vi "显示测试结果-左上角-拍照螺杆.vi"(8 "显示坐标":cluster{dbl, "Numeric":dbl}[](array[cluster])=[{100.0, "Numeric"=300.0}, {100.0, "Numeric"=400.0}, {100.0, "Numeric"=500.0}, {100.0, "Numeric"=600.0}, {100.0, "Numeric"=700.0}, {100.0, "Numeric"=800.0}, {100.0, "Numeric"=900.0}, {100.0, "Numeric"=1000.0}, {100.0, "Numeric"=1100.0}], 9 "量测项目名称":string[](array[string]), 10 "显示数据":dbl[](array[numeric]), 11 "Img输入":T1) -> ()   [LabVIEW 2014]
uses:
  <vilib>/vision/Image Controls.llb/IMAQ Image.ctl
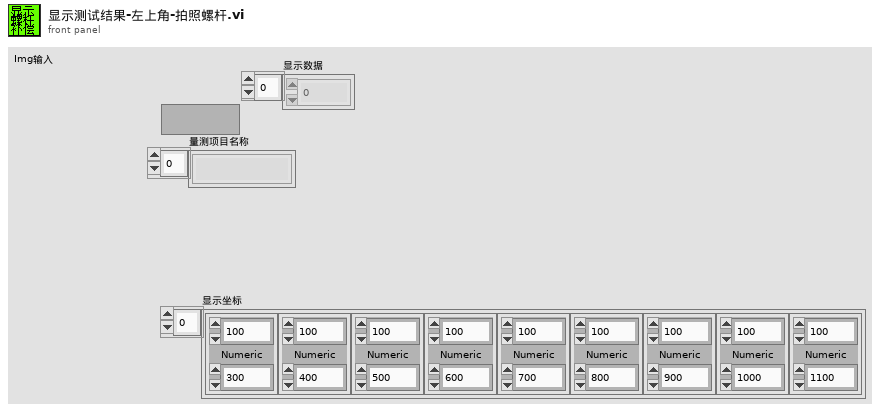
[diagram p1: front panel]
types:
  T1 = typedef "IMAQ Image.ctl" = refnum<image>
  T2 = cluster{"Desired Font (Application)":enum16{"User-specified Font", "Application Font", "System Font", "Dialog Font"}, "[User-specified Font]":cluster{"Font Name":string, "Size":i16, "Strikeout?":bool, "Italic?":bool, "Underline?":bool, "Outline?":bool, "Shadow?":bool, "Bold?":bool, "Rotation Angle":dbl}, "Horizontal Alignment":i16, "Vertical Alignment":i16}
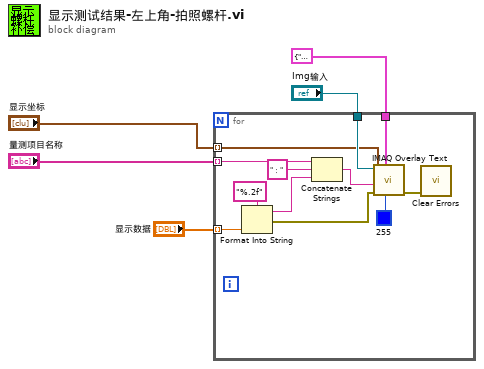
[diagram p0: block diagram]
diagram:
  n1 = for {
    tunnel: "Img输入" -> [w17]
    tunnel: "显示数据" -> [w16] mode=indexing
    tunnel: "显示坐标" -> [w15] mode=indexing
    tunnel: T2 {"Desired Font (Application)"=enum."User-specified Font", "[User-specified Font]"={"Font Name"="", "Size"=80, "Strikeout?"=FALSE, "Italic?"=FALSE, "Underline?"=FALSE, "Outline?"=FALSE, "Shadow?"=FALSE, "Bold?"=FALSE, "Rotation Angle"=0.0}, "Horizontal Alignment"=0, "Vertical Alignment"=0} ("Font, Size & Style") -> [w14]
    tunnel: "量测项目名称" -> [w10] mode=indexing
    n2 = Format Into String(format string="%.2f" ("格式字符串"), w16) -> (resulting string=w8:string, error out=w12:errorcluster)  [unwired: 2 in]
    n3 = Concatenate Strings(w10, "：" ("字符串"), w8) -> (w9:string)
    n4 = call "IMAQ Overlay Text"("Text Color (black)"=u32 255, "Font, Size & Style"=w14, "error in (no error)"=w12, "String"=w9, "Origin"=w15, "Image"=w17) -> ("error out"=w11:errorcluster)  [unwired: 4 in, 1 out]
    n5 = call <vilib>:"Clear Errors.vi"("error in (no error)"=w11) -> ()  [unwired: 5 in, 2 out]
  }
